vi "Change Laser Rep Rate.vi"(8 "error in":errorcluster, 11 "tCRD in":refnum<class "tCRD.lvclass">) -> (0 "error out":errorcluster, 3 "tCRD out":refnum<class "tCRD.lvclass">)   [LabVIEW 2015, in "tCRD.lvclass"]
doc: "Change the rate at which we modulate the laser. Make sure to pause the digitizer first before changing the modulation and restart it when we have reset the rep rate."
uses:
  tCRD.lvclass
  tCRD.lvclass/tCRD.ctl
  Reusable/Instrument/Instrument.lvclass/Instrument.ctl
  Reusable/Instrument/Write Restart Requested_.vi
  <vilib>/Utility/error.llb/Error Cluster From Error Code.vi
  <vilib>/rvi/errors/niLvFpgaAdjustHostInterfaceError.vi
  <vilib>/rvi/interface/nirviReadWriteControl/nirviReadWriteControl.xnode
  tFPGA Ref.ctl
  FPGA Bitfiles/FPGAServerwLRS.lvbitx
  <vilib>/rvi/interface/nirviMethod/nirviMethod.xnode
  NiFpgaLv.dll
  <vilib>/FPGAPlugInAG/sbRIO-9636/niLvFpga_ReadFifo_sbRIO-9636.vi
  <vilib>/rvi/errors/niLvFpgaMergeErrorWithErrorCode.vi
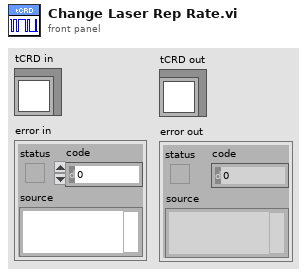
[diagram p1: front panel]
types:
  T1 = typedef "tCRD.lvclass/tFPGA Ref.ctl" = refnum<k20>
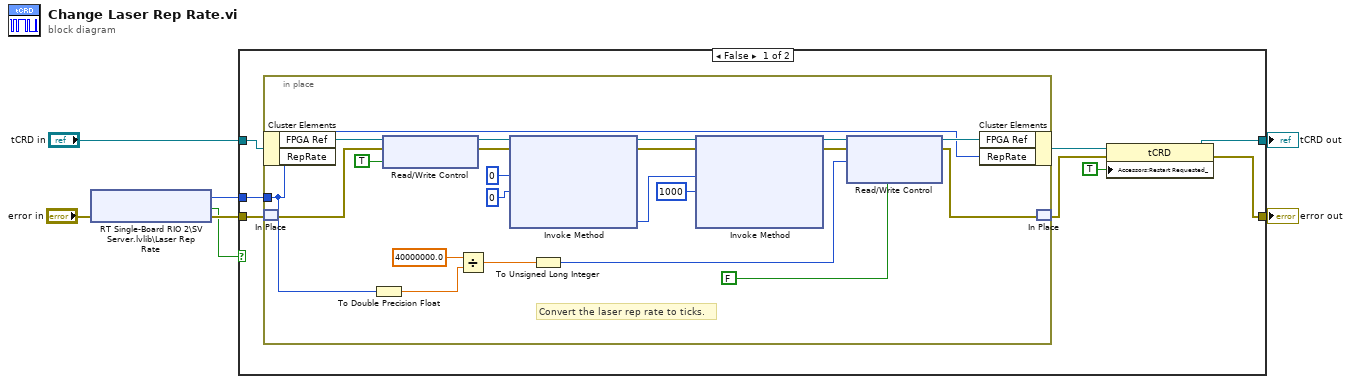
[diagram p0: block diagram]
diagram:
  n1 = shared-variable "RT Single-Board RIO 2\\SV Server.lvlib\\Laser Rep Rate"(error in="error in") -> (w2:u16, error out=w3:errorcluster, w1:bool)  [unwired: 1 in]
  n2 = case shown="False" w1 {
    tunnel: "tCRD in" -> [w15 w38]
    tunnel: [w11 w38] -> w6
    tunnel: [w10 w37] -> w5
    tunnel: w3 -> [w14 w37]
    tunnel: w2 -> [w13 _]
    frame False {
      n3 = in-place {
        in-place-border: w13 -> [w24]
        # "Convert the laser rep rate to ticks."
        n4 = in-place-cluster #1(w15) -> ("FPGA Ref"=w29:T1)  [unwired: 1 out]
        n5 = in-place-match #2(w14) -> (w26:errorcluster)
        n6 = To Double Precision Float(number=w24) -> (double precision float=w32:dbl)
        n7 = xnode "Read/Write Control"("FPGA VI Reference In"=w29, "error in"=w26, "Pause Digitizer"=TRUE) -> ("FPGA VI Reference Out"=w35:T1, "error out"=w34:errorcluster)
        n8 = Divide(x=40000000.0, y=w32) -> (x/y=w30:dbl)
        n9 = xnode "Invoke Method"("FPGA VI Reference In"=w35, "error in"=w34, "Number of Elements"=u32 0, "Timeout (ms)"=0) -> ("FPGA VI Reference Out"=w21:T1, "error out"=w19:errorcluster, "Elements Remaining"=w18:u32)  [unwired: 1 out]
        n10 = To Unsigned Long Integer(number=w30) -> (unsigned 32bit integer=w25:u32)
        n11 = xnode "Invoke Method"("FPGA VI Reference In"=w21, "error in"=w19, "Number of Elements"=w18, "Timeout (ms)"=1000) -> ("FPGA VI Reference Out"=w20:T1, "error out"=w16:errorcluster)  [unwired: 2 out]
        n12 = xnode "Read/Write Control"("FPGA VI Reference In"=w20, "error in"=w16, "Cylce (ticks)"=w25, "Pause Digitizer"=FALSE) -> ("FPGA VI Reference Out"=w28:T1, "error out"=w27:errorcluster)
        n13 = in-place-cluster #1("FPGA Ref"=w28, "RepRate"=w24) -> (w12:refnum<class "tCRD.lvclass">)
        n14 = in-place-match #2(w27) -> (w9:errorcluster)
      }
      n15 = property class="tCRD"(reference=w12, error in=w9, "Accessors:Restart Requested_"=TRUE ("Restart Requested_")) -> (reference out=w11:refnum<class "tCRD.lvclass">, error out=w10:errorcluster)
    }
    frame True {
    }
  }
  "tCRD out" <- w6
  "error out" <- w5
